vi "CAN Monitor Init.vi"(9 "CAN Ports":string[](array[string]), 10 "CAN.BusLoad.Settings":T3[](array[typedef]), 11 "Data Access Engine in":refnum<class "Data Access Engine.lvclass">) -> (0 "error out":errorcluster, 3 "CAN Runtime Data":T1[](array[typedef]))   [LabVIEW 2018, in "NI-XNET Monitor Engine.lvlib"]
uses:
  NI-XNET Monitor Engine.lvlib
  Shared/BusLoad.Settings.ctl
  typedefs/CANBus.Settings.ctl
  Bus Load/CANBus/CANBus_Load_Calculator.lvclass
  <vilib>/NI/NIVS Inline Async API/_Data Access Engine/Data Access Engine/Types/Write.DVR.ctl
  <vilib>/NI/NIVS Inline Async API/_Data Access Engine/Access Type Classes/Write/Write.lvclass
  <vilib>/NI/NIVS Inline Async API/_Data Access Engine/Data Access Engine/Data Access Engine.lvclass
  <vilib>/NI/NIVS Inline Async API/_Data Access Engine/Data Access Engine/Methods/Write.Lookup.vi
  Bus Load/XNET-Bus-Load-Calculator.lvlib
  Shared/NI-XNET Monitor Shared.lvlib
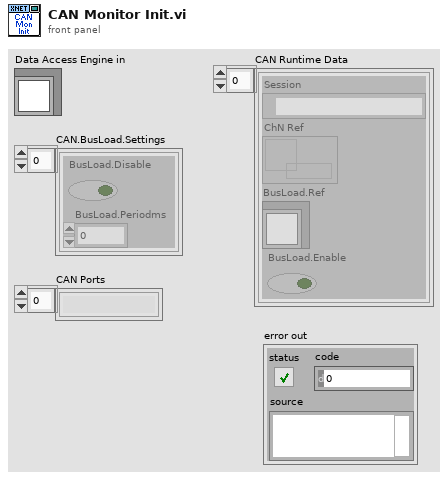
[diagram p1: front panel]
types:
  T1 = typedef "NI-XNET Monitor Engine.lvlib/CANBus.Settings.ctl" = cluster{"Session":refnum<k21>, "ChN Ref":T2, "BusLoad.Ref":refnum<class "CANBus_Load_Calculator.lvclass">, "BusLoad.Enable":bool}
  T2 = typedef "Data Access Engine.lvlib/Data Access Engine.lvclass/Write.DVR.ctl" = refnum<data-value>
  T3 = typedef "NI-XNET Monitor Shared.lvlib/BusLoad.Settings.ctl" = cluster{"BusLoad.Disable":bool, "BusLoad.Periodms":u32}
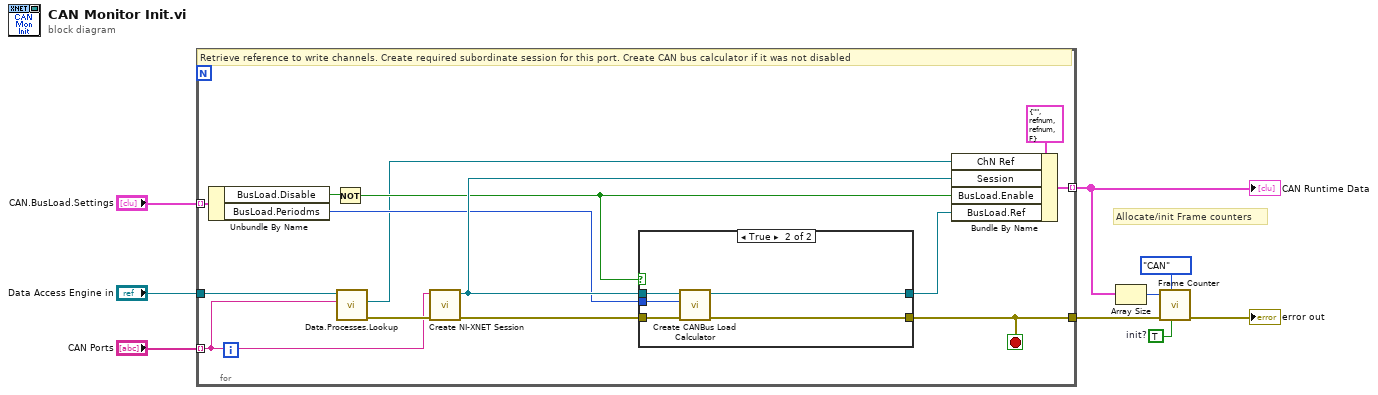
[diagram p0: block diagram]
diagram:
  w4 = TRUE  # init?
  # "Allocate/init Frame counters"
  n1 = for {
    tunnel: "CAN Ports" -> [w20] mode=indexing
    tunnel: "Data Access Engine in" -> [w22]
    tunnel: [w15] -> w7
    tunnel: [w18] -> w6 mode=indexing
    tunnel: "CAN.BusLoad.Settings" -> [w17] mode=indexing
    stop <- w15 stop-if-true
    # "Retrieve reference to write channels. Create required subordinate session for this port. Create CAN bus calculator if it was not disabled"
    n2 = Unbundle By Name(w17) -> ("BusLoad.Disable"=w14:bool, "BusLoad.Periodms"=w10:u32)
    n3 = Not(x=w14) -> (.not. x?=w12:bool)
    n4 = call-poly <vilib>:"Data.Processes.Lookup.vi"("Name"=w20, "Data Access API in"=w22) -> ("error out"=w21:errorcluster, "Ref"=w9:T2)  [unwired: 6 in, 2 out]
    n5 = call "Create NI-XNET Session.vi"("Error In"=w21, "NI-XNET Port In"=w20) -> ("Error Out"=w16:errorcluster, "Session out"=w13:refnum<k21>)  [unwired: 8 in]
    n6 = case shown="True" w12 {
      tunnel: w16 -> [w23 w28]
      tunnel: [w23 w27] -> w15
      tunnel: w13 -> [_ w26]
      tunnel: [_ w25] -> w11
      tunnel: w10 -> [_ w24]
      frame False {
      }
      frame True {
        n7 = call "Create CANBus Load Calculator.vi"("error in (no error)"=w28, "Calculation Period (ms)"=w24, "XNET Session"=w26) -> ("error out"=w27:errorcluster, "CANBus Load Calculator"=w25:refnum<class "CANBus_Load_Calculator.lvclass">)  [unwired: 7 in]
      }
    }
    n8 = Bundle By Name(cluster=T1 {"Session"="", "ChN Ref"=refnum, "BusLoad.Ref"=refnum, "BusLoad.Enable"=FALSE} ("CANBus.Settings"), "ChN Ref"=w9, "Session"=w13, "BusLoad.Enable"=w12, "BusLoad.Ref"=w11) -> (w18:T1)
  }
  "error out" <- w7
  "CAN Runtime Data" <- w6
  n9 = Array Size(array=w6) -> (size(s)=w5:i32)
  n10 = call "Frame Counter.vi"("init? (F)"=w4, "bus type"=enum16{"CAN", "FlexRay", "LIN"}."CAN", "error in (no error)"=w7, "bus index (bus count for init)"=w5) -> ()  [unwired: 6 in, 2 out]
